vi "Read TCP Line with CRLF.vi"(0 "TCP Connection In":refnum<k5>, 7 "timeout ms (100)":i32=100, 11 "error in":errorcluster) -> (4 "TCP Connection Out":refnum<k5>, 8 "TCP Line":string, 15 "error out":errorcluster)   [LabVIEW 2011, in "ART2 Test Panel.lvlib"]
uses:
  ART2 Test Panel.lvlib
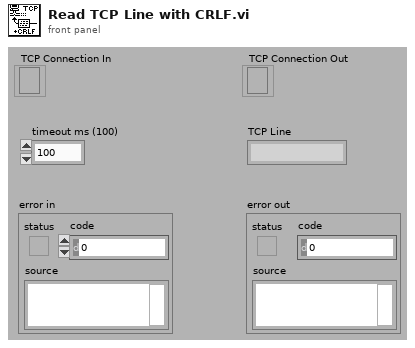
[diagram p1: front panel]
types:
  T1 = enum16{"Standard", "Buffered", "CRLF", "Immediate"}
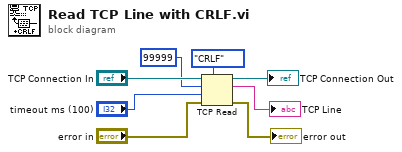
[diagram p0: block diagram]
diagram:
  n1 = TCP Read(connection ID="TCP Connection In", bytes to read=99999, error in (no error)="error in", 7:T1."CRLF" ("mode (standard)"), 9:"timeout ms (100)") -> (connection ID out=→"TCP Connection Out":refnum<k5>, data out=→"TCP Line":string, error out=→"error out":errorcluster)
